vi "Get Owning Path Default Value.vi"(0 "Scalar Path Group in":refnum<class "Scalar Path Group.lvclass">, 11 "error in (no error)":errorcluster) -> (4 "Scalar Path Group out":refnum<class "Scalar Path Group.lvclass">, 6 "Path":refnum<class "Path.lvclass">, 15 "error out":errorcluster)   [LabVIEW 2023, in "RFFixtureCharact.Public.lvlib" / "Scalar Path Group.lvclass"]
uses:
  Scalar Path Group.lvclass
  Common/Base Classes/Path/Path.lvclass
  Scalar Path/Scalar Path.lvclass
  C:/srd-semi-rfcal-software/AuxTools/STSRFFixtureCharactUtility/Source/Code Modules/Common/Base Classes/Path/Path.lvclass
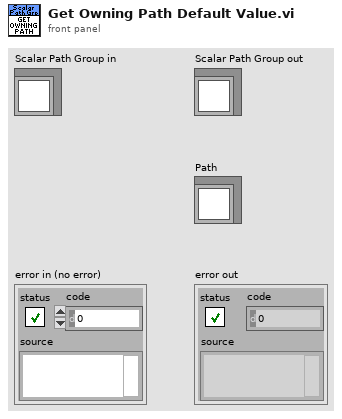
[diagram p1: front panel]
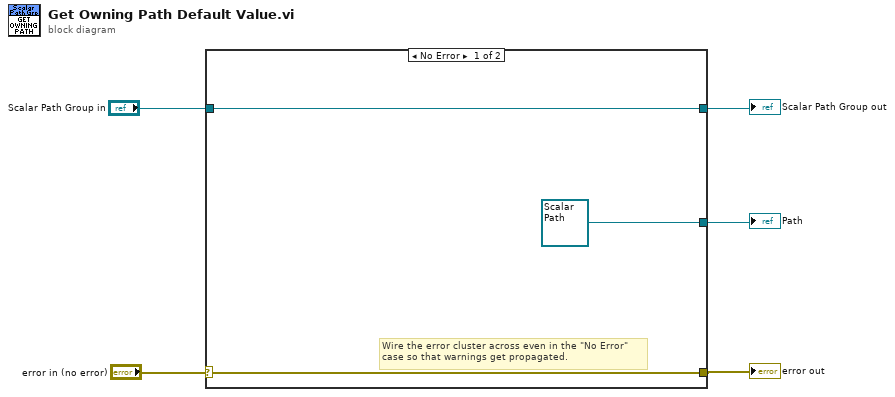
[diagram p0: block diagram]
diagram:
  n1 = case shown="No Error" "error in (no error)" {
    selector: "error in (no error)" -> [w7 w10]
    tunnel: [w7 w10] -> w1
    tunnel: [w8 w9] -> w3
    tunnel: "Scalar Path Group in" -> [w8 w9]
    tunnel: [refnum<class "Scalar Path.lvclass"> refnum ("Calibration Common.lvlib:Path.lvclass") _] -> w2
    frame No Error {
      # "Wire the error cluster across even in the \"No Error\"\ncase so that warnings get propagated."
    }
    frame Error {
    }
  }
  "error out" <- w1
  "Scalar Path Group out" <- w3
  "Path" <- w2
